vi "Main VI.vi"() -> ()   [LabVIEW 2022 SP3]
panel:
  out "Waveform Chart":dynamicdata(graph)
  out "SampClk.Rate Indicator":dbl
  in  "File Name":string
  in  "Tab Control":enum32{"Test Firing", "Cold Flow Rig"}(tab)
  in  "Collect Data?":bool=TRUE caption="Enable"
  out "Filename Out":path
  in  "Cold Flow - Collect data?":bool=TRUE caption="Enable"
  out "Cold Flow - Filename Out":path caption="Filename Out"
  out "error out":errorcluster
  in  "stop":bool
  in  "number of samples":i32=100
  in  "File Format":string
  in  "Data Collection Folder":path
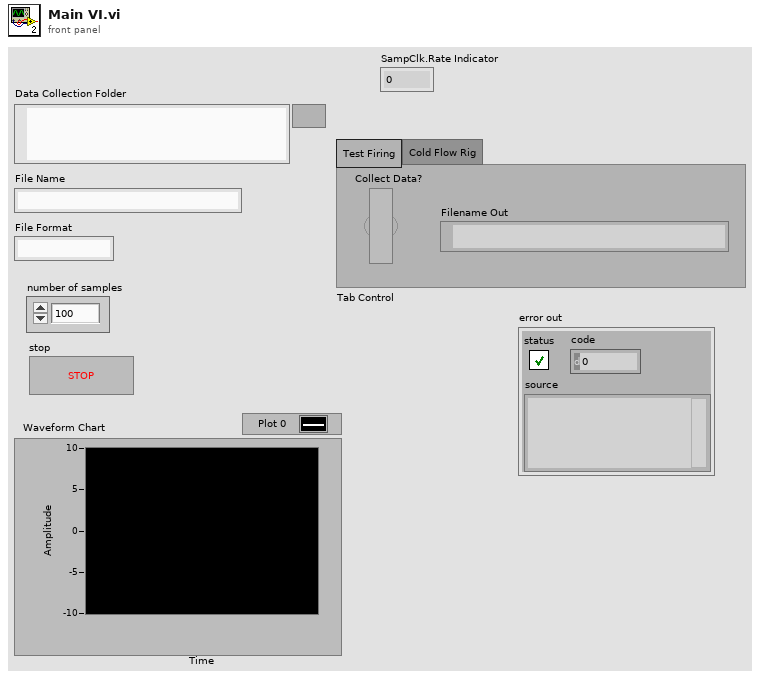
[diagram p1: front panel]
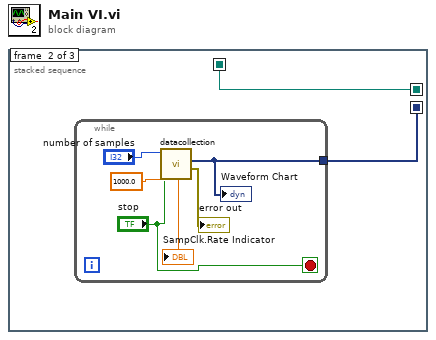
[diagram p0: block diagram]
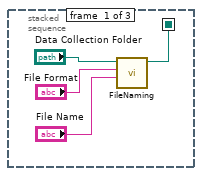
[diagram p2: hidden frame]
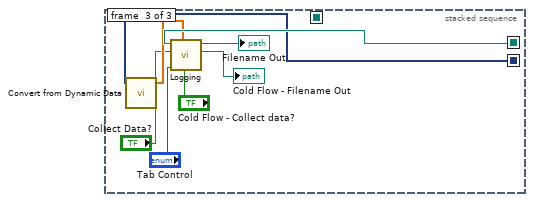
[diagram p3: hidden frame]
diagram:
  n1 = stacked-sequence {
    seq-local: [w1 _ _] -> [_ w6 _]
    seq-local: [_ w6 _] -> [_ _ w20]
    seq-local: [_ w5 _] -> [_ _ w19]
    frame #0 {
      n2 = call "FileNaming.vi"("File Name Out"="File Name", "File Format"="File Format", "Data Collection Folder"="Data Collection Folder") -> ("path"=w1:path)  [unwired: 8 in]
    }
    frame #1 {
      n3 = while {
        tunnel: [w8] -> w5
        stop <- "stop" stop-if-true
        n4 = call "datacollection.vi"("stop"="stop", "rate"=1000.0, "samples per channel"="number of samples") -> ("error out"=→"error out":errorcluster, "All Sensors"=w8:dynamicdata, "SampClk.Rate Indicator"=→"SampClk.Rate Indicator":dbl)  [unwired: 5 in, 1 out]
        "Waveform Chart" <- w8
      }
    }
    frame #2 {
      n5 = call "Convert from Dynamic Data"("Dynamic Data Type"=w19) -> ("Array"=w18:dbl[])  [unwired: 3 in]
      n6 = call "Logging.vi"("Signals in (Array DBL)"=w18, "Tab Control"="Tab Control", "Cold Flow - Collect data?"="Cold Flow - Collect data?", "Collect Data?"="Collect Data?", "Filename"=w20) -> ("Cold Flow - Filename Out"=→"Cold Flow - Filename Out":path, "Filename Out"=→"Filename Out":path)  [unwired: 5 in]
    }
  }
